vi "Add Elements to Meas Plugin UI - Single Converter.vi"(11 "error in":errorcluster) -> (15 "error out":errorcluster)   [LabVIEW 2021, in "Converter.lvlib"]
uses:
  Converter.lvlib
  Path Functions/Path Functions.lvlib
  Converter Reusables/Converter Reusables.lvlib
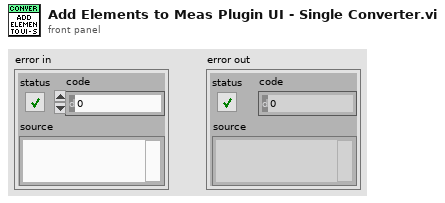
[diagram p1: front panel]
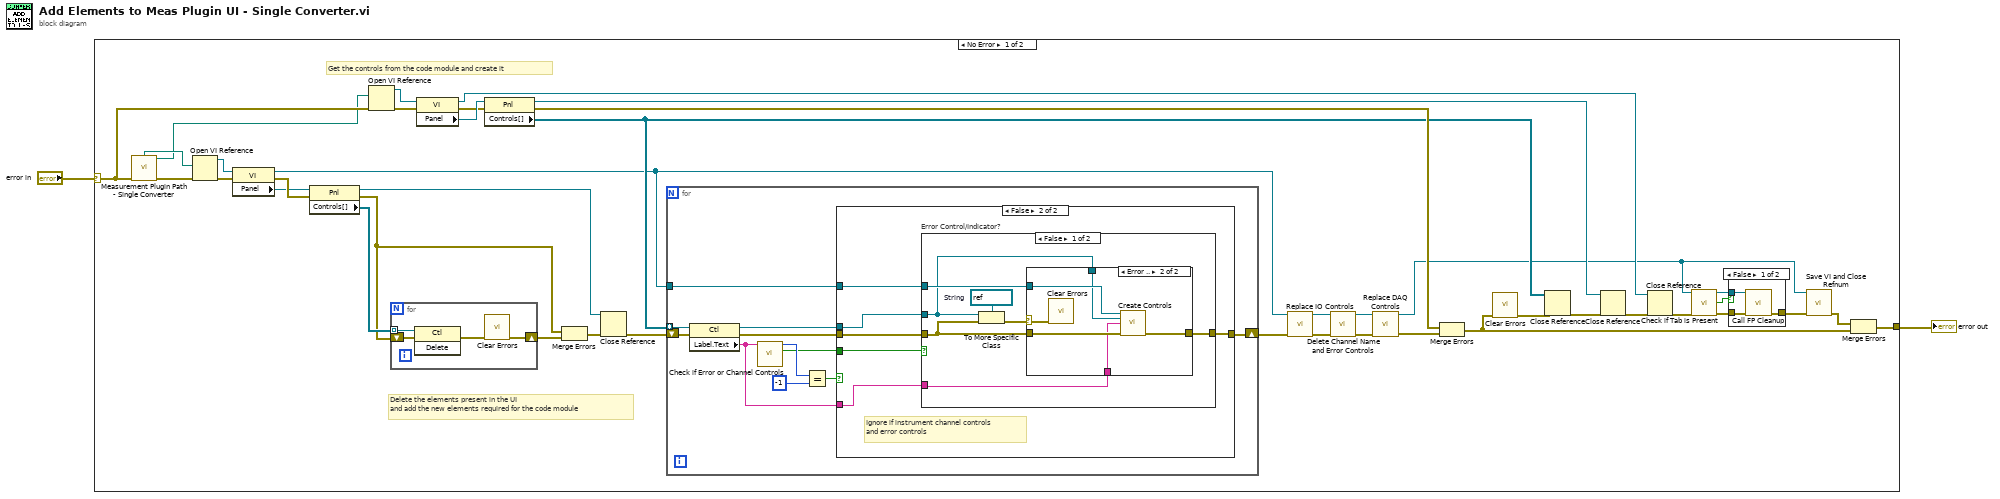
[diagram p0: block diagram]
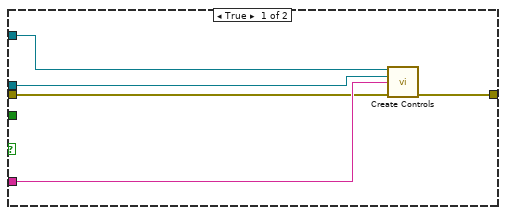
[diagram p3: hidden frame]
diagram:
  n1 = case shown="No Error" "error in" {
    selector: "error in" -> [w29 w89]
    tunnel: [w33 w89] -> w2
    frame No Error {
      # "Get the controls from the code module and create it"
      # "Delete the elements present in the UI\nand add the new elements required for the code module"
      n2 = call "Measurement Plugin Path - Single Converter.vi"("error in"=w29) -> ("measurement ui"=w31:path, "new code module"=w12:path, "error out"=w43:errorcluster)  [unwired: 2 in, 10 out]
      n3 = Open VI Reference(vi path=w31, error in (no error)=w43) -> (vi reference=w21:refnum<vi>, error out=w42:errorcluster)  [unwired: 4 in]
      n4 = property class="VI"(reference=w21, error in=w42) -> (reference out=w25:refnum<vi>, error out=w41:errorcluster, "Panel"=w27:refnum<vi>)
      n5 = property class="Pnl"(reference=w27, error in=w41) -> (reference out=w26:refnum<vi>, error out=w13:errorcluster, "Controls[]"=w40:refnum<vi>[])
      n6 = Open VI Reference(vi path=w12, error in (no error)=w29) -> (vi reference=w19:refnum<vi>, error out=w35:errorcluster)  [unwired: 4 in]
      n7 = for {
        tunnel: w40 -> [w88] mode=indexing
        shift-right: [w85] -> w39
        shift-left: w13 -> [w87]
        n8 = invoke class="Ctl" method="Delete"(reference=w88, error in=w87) -> (error out=w86:errorcluster)  [unwired: 1 in, 2 out]
        n9 = call <vilib>:"Clear Errors.vi"("error in (no error)"=w86) -> ("error out"=w85:errorcluster)  [unwired: 5 in, 1 out]
      }
      n10 = property class="VI"(reference=w19, error in=w35) -> (reference out=w18:refnum<vi>, error out=w34:errorcluster, "Panel"=w36:refnum<vi>)
      n11 = property class="Pnl"(reference=w36, error in=w34) -> (reference out=w17:refnum<vi>, error out=w38:errorcluster, "Controls[]"=w37:refnum<vi>[])
      n12 = Merge Errors(w13, w39) -> (w14:errorcluster)
      n13 = Close Reference(reference=w26, error in (no error)=w14) -> (error out=w28:errorcluster)
      n14 = for {
        tunnel: w25 -> [w58]
        tunnel: w37 -> [w56] mode=indexing
        shift-right: [w57] -> w24
        shift-left: w28 -> [w48]
        n15 = property class="Ctl"(reference=w56, error in=w48) -> (reference out=w54:refnum<vi>, error out=w53:errorcluster, "Label.Text"=w55:string)
        n16 = call "Check if Error or Channel Controls.vi"("label.text"=w55) -> ("error?"=w49:bool, "offset past match"=w52:i32)  [unwired: 9 in]
        n17 = Equal?(x=w52, y=-1) -> (x = y?=w50:bool)
        n18 = case shown="False" w50 {
          tunnel: w58 -> [w63 w66]
          tunnel: [w62 w64] -> w57
          tunnel: w54 -> [w60 w69]
          tunnel: w53 -> [w59 w68]
          tunnel: w55 -> [w61 w65]
          tunnel: w49 -> [_ w67]
          frame True {
            n19 = call "Create Controls.vi"("vi in"=w63, "ctl refnum"=w60, "control label"=w61, "error in"=w59) -> ("error out"=w62:errorcluster)  [unwired: 11 in]
          }
          frame False {
            # "Ignore if instrument channel controls\nand error controls"
            n20 = case "Error Control/Indicator?" shown="False" w67 {
              tunnel: w69 -> [w72 _]
              tunnel: w68 -> [w75 w84]
              tunnel: w66 -> [w73 _]
              tunnel: w65 -> [w71 _]
              tunnel: [w70 w84] -> w64
              frame False {
                w76 = refnum<vi> refnum  # String
                n21 = To More Specific Class(target class=w76, reference=w72, error in=w75) -> (error out=w74:errorcluster)  [unwired: 1 out]
                n22 = case shown="Error .." w74 {
                  selector: w74 -> [_ w78]
                  tunnel: w75 -> [w77 w83]
                  tunnel: w73 -> [_ w82]
                  tunnel: w72 -> [_ w81]
                  tunnel: w71 -> [_ w80]
                  tunnel: [w77 w79] -> w70
                  frame No Error {
                  }
                  frame Error {
                    n23 = call <vilib>:"Clear Errors.vi"("error in (no error)"=w78) -> ()  [unwired: 5 in, 2 out]
                    n24 = call "Create Controls.vi"("vi in"=w82, "ctl refnum"=w81, "control label"=w80, "error in"=w83) -> ("error out"=w79:errorcluster)  [unwired: 11 in]
                  }
                }
              }
              frame True {
              }
            }
          }
        }
      }
      n25 = call "Replace IO Controls.vi"("vi in"=w25, "error in"=w24) -> ("vi out"=w23:refnum<vi>, "error out"=w22:errorcluster)  [unwired: 12 in]
      n26 = call "Delete Channel Name and Error Controls.vi"("vi in"=w23, "error in"=w22) -> ("vi out"=w7:refnum<vi>, "error out"=w4:errorcluster)  [unwired: 12 in]
      n27 = call "Replace DAQ Controls.vi"("vi in"=w7, "error in"=w4) -> ("vi out"=w6:refnum<vi>, "error out"=w5:errorcluster)  [unwired: 12 in]
      n28 = Merge Errors(w38, w5) -> (w3:errorcluster)
      n29 = call <vilib>:"Clear Errors.vi"("error in (no error)"=w3) -> ("error out"=w32:errorcluster)  [unwired: 5 in, 1 out]
      n30 = Close Reference(reference=w37, error in (no error)=w32) -> (error out=w15:errorcluster)
      n31 = Close Reference(reference=w17, error in (no error)=w15) -> (error out=w16:errorcluster)
      n32 = Close Reference(reference=w18, error in (no error)=w16) -> (error out=w10:errorcluster)
      n33 = call "Check if Tab is Present.vi"("vi in"=w6, "error in"=w10) -> ("vi out"=w11:refnum<vi>, "tab present?"=w8:bool, "error out"=w9:errorcluster)  [unwired: 11 in]
      n34 = case shown="False" w8 {
        tunnel: [w46 w47] -> w20
        tunnel: w11 -> [w45 _]
        tunnel: w9 -> [w44 w47]
        frame False {
          n35 = call "Call FP Cleanup.vi"("vi"=w45, "error in"=w44) -> ("error out"=w46:errorcluster)  [unwired: 13 in]
        }
        frame True {
        }
      }
      n36 = call "Save VI and Close Refnum.vi"("vi refnum"=w6, "error in"=w20) -> ("error out"=w30:errorcluster)  [unwired: 13 in]
      n37 = Merge Errors(w30, w3) -> (w33:errorcluster)
    }
    frame Error {
    }
  }
  "error out" <- w2
